vi "destroyQueueTcpClientFromDds.vi"(8 "error in (no error)":errorcluster, 11 "TcpServerTel in":refnum<class "TcpServerTel.lvclass">) -> (0 "error out":errorcluster, 3 "TcpServerTel out":refnum<class "TcpServerTel.lvclass">)   [LabVIEW 2018, in "TcpServerTel.lvclass"]
doc: "Destroy queueTcpClientFromDds reference."
uses:
  TcpServerTel.lvclass
  TcpServerTel.lvclass/TcpServerTel.ctl
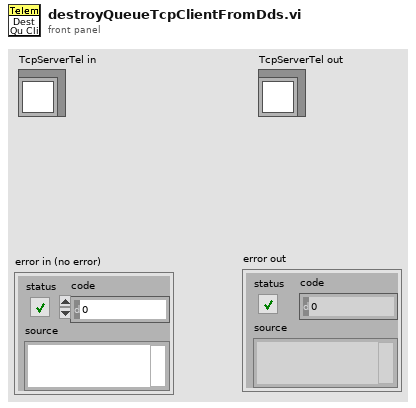
[diagram p1: front panel]
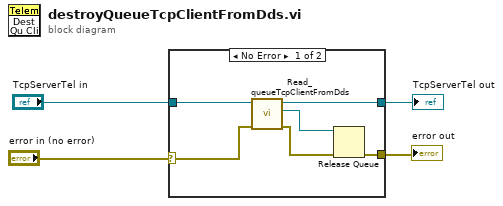
[diagram p0: block diagram]
diagram:
  n1 = case shown="No Error" "error in (no error)" {
    selector: "error in (no error)" -> [w5 w11]
    tunnel: "TcpServerTel in" -> [w10 w12]
    tunnel: [w7 w12] -> w3
    tunnel: [w6 w11] -> w2
    frame No Error {
      n2 = call "Read_queueTcpClientFromDds.vi"("error in (no error)"=w5, "TcpServerTel in"=w10) -> ("error out"=w8:errorcluster, "queueTcpClientFromDds"=w9:refnum<queue>, "TcpServerTel out"=w7:refnum<class "TcpServerTel.lvclass">)  [unwired: 7 in]
      n3 = Release Queue(queue=w9, error in (no error)=w8) -> (error out=w6:errorcluster)  [unwired: 1 in, 2 out]
    }
    frame Error {
    }
  }
  "error out" <- w2
  "TcpServerTel out" <- w3
